vi "Auto_Range.vi"(0 "VisaCluster":T1, 7 "Auto_Range":bool, 11 "error in (no error)":errorcluster) -> (4 "VisaCluster":T1, 6 "Answer":string, 8 "Auto":bool=TRUE, 10 "Display":string, 15 "error out":errorcluster)   [LabVIEW 2014, in "FH 55.lvlib"]
doc: "This VI sets the Auto Range ON or OFF. \n\nDurch das VI Auto_Range kann die automatische Messbereichswahl eingeschaltet werden. Auto kann nicht zusammen mit den Funktionen Peak und Max./Min. verwendet werden. Auch darf Auto nicht zur Messung kleiner Magnetfelder bei großem Hintergrundfeld verwendet werden."
uses:
  FH 55.lvlib
  TypeDef/VisaCluster.ctl
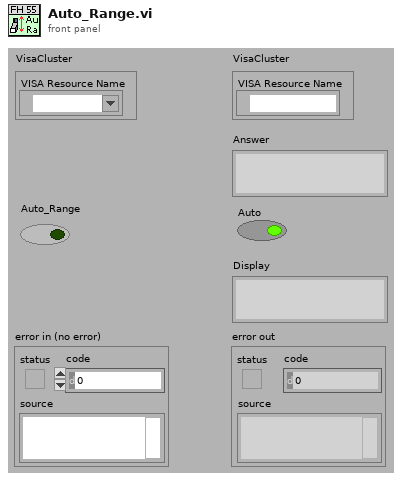
[diagram p1: front panel]
types:
  T1 = typedef "FH 55.lvlib/VisaCluster.ctl" = cluster{"VISA Resource Name":refnum<visa-resource-name>}
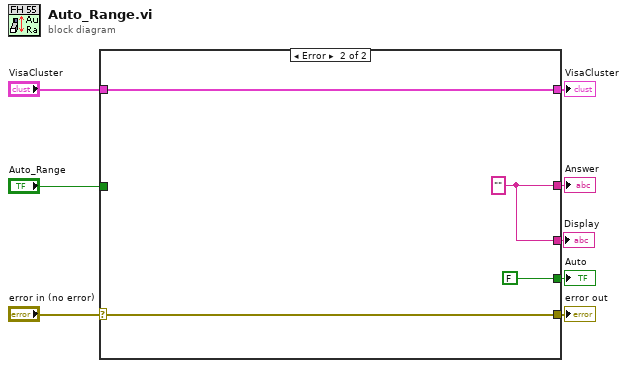
[diagram p0: block diagram]
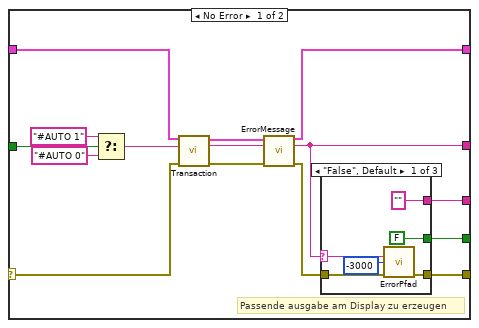
[diagram p2: hidden frame]
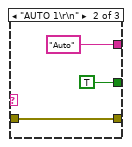
[diagram p3: hidden frame]
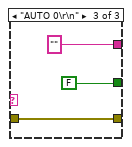
[diagram p4: hidden frame]
diagram:
  n1 = case shown="Error" "error in (no error)" {
    selector: "error in (no error)" -> [w17 w38]
    tunnel: "VisaCluster" -> [w19 w39]
    tunnel: "Auto_Range" -> [w23 _]
    tunnel: [w20 w39] -> w4
    tunnel: [w10 w38] -> w6
    tunnel: [w13 w37] -> w5
    tunnel: [w12 w37] -> w2
    tunnel: [w9 FALSE] -> w1
    frame No Error {
      # "Passende ausgabe am Display zu erzeugen"
      n2 = Select(t="#AUTO 1", s=w23, f="#AUTO 0") -> (s? t:f=w18:string)
      n3 = call "Transaction.vi"("VisaCluster"=w19, "Command"=w18, "error in (no error)"=w17) -> ("VisaCluster"=w14:T1, "Answer"=w15:string, "error out"=w16:errorcluster)  [unwired: 9 in, 1 out]
      n4 = call "ErrorMessage.vi"("VisaCluster"=w14, "Message In"=w15, "error in (no error)"=w16) -> ("VisaCluster"=w20:T1, "Message Out"=w13:string, "error out"=w11:errorcluster)  [unwired: 10 in]
      n5 = case shown="\"False\", Default" w13 {
        selector: w13 -> [w26 _ _]
        tunnel: ["" "Auto" ""] -> w12
        tunnel: w11 -> [w28 w31 w34]
        tunnel: [w27 w31 w34] -> w10
        tunnel: [FALSE TRUE FALSE] -> w9
        frame "False", Default {
          n6 = call "ErrorPfad.vi"("Message In"=w26, "Numeric"=-3000, "error in (no error)"=w28) -> ("error out"=w27:errorcluster)  [unwired: 11 in, 1 out]
        }
        frame "AUTO 1\r\n" {
        }
        frame "AUTO 0\r\n" {
        }
      }
    }
    frame Error {
      w37 = ""
    }
  }
  "error out" <- w6
  "Answer" <- w5
  "VisaCluster" <- w4
  "Display" <- w2
  "Auto" <- w1
